vi "Denoising.vi"(0 "Higher Cut-Off\nfor Highpass Filter":dbl=1.0, 1 "Lower Cut-Off\nfor Lowpass Filter":dbl=70.0, 2 "Array in":dbl[][](array[numeric]), 3 "Lower Cut-Off\nfor Notch Filter":dbl=45.0 caption="Lower Cut-Off", 4 "Upper Cut-Off\nfor Notch Filter":dbl=60.0 caption="Upper Cut-Off", 5 "Sampling Frequency\nfor  Bandpass Filtering":dbl=512.0, 8 "Absolute Data":bool) -> (7 "Array out":dbl[][](array[numeric]))   [LabVIEW 2023]
uses:
  <vilib>/Analysis/3filter.llb/Filter Passband Type.ctl
  <vilib>/Analysis/NI_AALBase.lvlib
panel:
  out "Notch Filtered Signal":dbl
  out "Notch Filtered Waveform":dynamicdata(graph) caption="Filtered Signal"
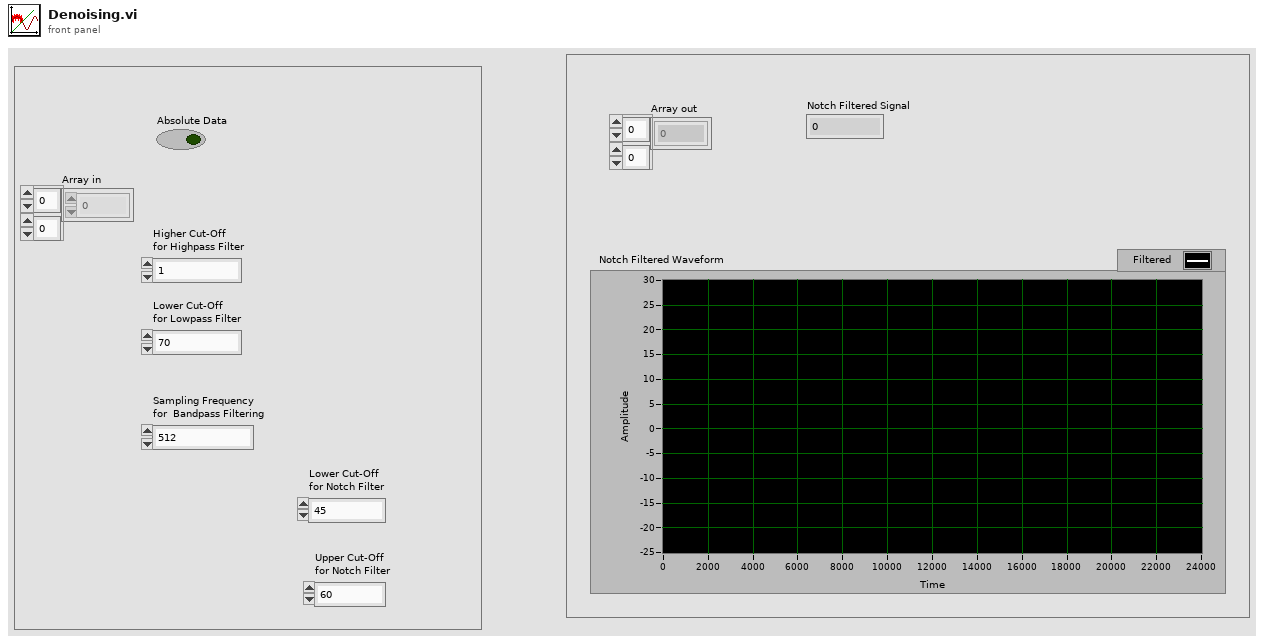
[diagram p1: front panel]
types:
  T1 = typedef "NI_AALBase.lvlib/Filter Passband Type.ctl" = enum32{"Lowpass", "Highpass", "Bandpass", "Bandstop"}
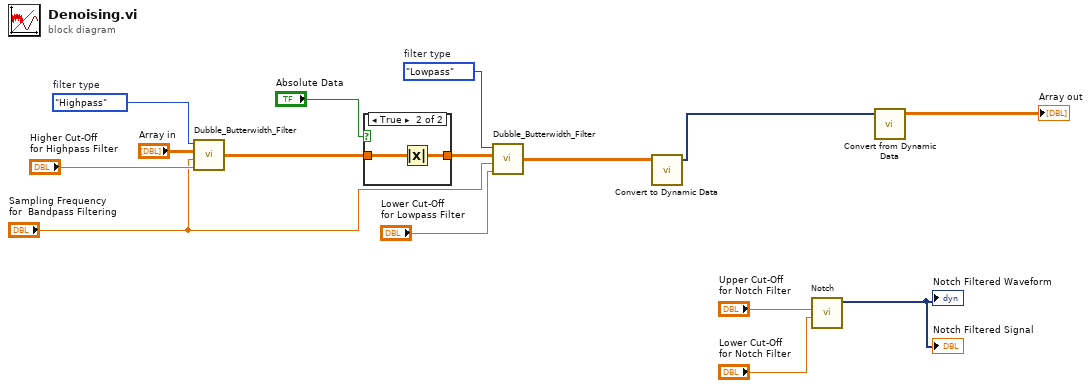
[diagram p0: block diagram]
diagram:
  w7 = Filter_Passband_Type."Lowpass"  # filter type
  w8 = Filter_Passband_Type."Highpass"  # filter type
  n1 = call "Dubble_Butterwidth_Filter.vi"("Higher Cut-Off"="Higher Cut-Off\nfor Highpass Filter", "sampling freq: fs"="Sampling Frequency\nfor  Bandpass Filtering", "Array in"="Array in", "filter type"=w8) -> ("Array out"=w13:dbl[][])
  n2 = case shown="True" "Absolute Data" {
    tunnel: w13 -> [w16 w18]
    tunnel: [w16 w17] -> w14
    frame False {
    }
    frame True {
      n3 = Absolute Value(x=w18) -> (abs(x)=w17:dbl[][])
    }
  }
  n4 = call "Dubble_Butterwidth_Filter.vi"("Higher Cut-Off"="Lower Cut-Off\nfor Lowpass Filter", "sampling freq: fs"="Sampling Frequency\nfor  Bandpass Filtering", "Array in"=w14, "filter type"=w7) -> ("Array out"=w5:dbl[][])
  n5 = call "Convert to Dynamic Data"("2D Array"=w5) -> ("Dynamic Data Type"=w2:dynamicdata)  [unwired: 3 in]
  n6 = call "Notch"("Lower Cut-Off"="Lower Cut-Off\nfor Notch Filter", "Upper Cut-Off"="Upper Cut-Off\nfor Notch Filter") -> ("Filtered Signal"=→"Notch Filtered Waveform" →"Notch Filtered Signal":dynamicdata)  [unwired: 2 in, 7 out]
  n7 = call "Convert from Dynamic Data"("Dynamic Data Type"=w2) -> ("Array"=→"Array out":dbl[][])  [unwired: 3 in]
